vi "VISA_Query.vi"(8 "Byte Count":u32=9, 10 "VISA Refnum in":refnum<visa-resource-name>="COM6") -> (0 "chamber":dbl, 1 "Chamber Pressure (mbar)":string, 2 "Scroll Pump Pressure (mbar)":string, 3 "VISA Refnum out":refnum<visa-resource-name>, 7 "scroll pump":dbl)   [LabVIEW 2016]
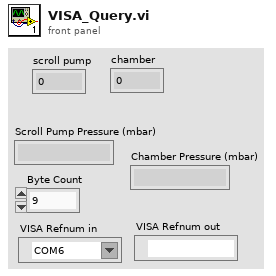
[diagram p1: front panel]
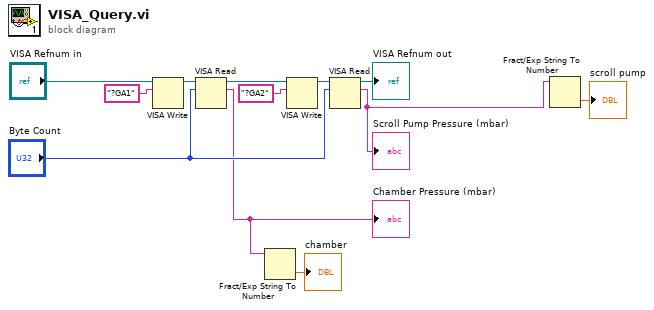
[diagram p0: block diagram]
diagram:
  n1 = VISA Write(VISA resource name="VISA Refnum in", write buffer="?GA1") -> (VISA resource name out=w8:refnum<visa-resource-name>)  [unwired: 1 in, 2 out]
  n2 = VISA Read(VISA resource name=w8, byte count="Byte Count") -> (VISA resource name out=w10:refnum<visa-resource-name>, read buffer=w2:string)  [unwired: 1 in, 2 out]
  "Chamber Pressure (mbar)" <- w2
  n3 = Fract/Exp String To Number(string=w2) -> (number=→"chamber":dbl)  [unwired: 3 in, 1 out]
  n4 = VISA Write(VISA resource name=w10, write buffer="?GA2") -> (VISA resource name out=w9:refnum<visa-resource-name>)  [unwired: 1 in, 2 out]
  n5 = VISA Read(VISA resource name=w9, byte count="Byte Count") -> (VISA resource name out=→"VISA Refnum out":refnum<visa-resource-name>, read buffer=w4:string)  [unwired: 1 in, 2 out]
  "Scroll Pump Pressure (mbar)" <- w4
  n6 = Fract/Exp String To Number(string=w4) -> (number=→"scroll pump":dbl)  [unwired: 3 in, 1 out]
